vi "launch_automatic.vi"(5 "waitgroup":T5, 7 "references":T3, 8 "error in (no error)":errorcluster, 10 "data":T1, 11 "vi_reference":variant) -> (0 "error out":errorcluster)   [LabVIEW 2015, in "lv-recipe-machine.lvlib"]
uses:
  lv-recipe-machine.lvlib
  <userlib>/antonio-alexander/lv-waitgroup/public/_controls/api_waitgroup.ctl
  public/_controls/references.ctl
  public/_controls/input.ctl
  public/_controls/input_command.ctl
  public/_controls/output.ctl
  public/_controls/data.ctl
  public/_controls/configuration.ctl
  public/_controls/recipe_data.ctl
  public/_controls/mode.ctl
  public/_controls/manual_state.ctl
  public/_controls/automatic_state.ctl
  public/_controls/recipe_step.ctl
  public/_controls/change.ctl
  public/_controls/status.ctl
  _controls/automatic_vi_variant_data.ctl
  public/_controls/vi_reference_automatic_step.ctl
  public/_controls/vi_reference_criteria.ctl
  public/_controls/vi_reference_transition.ctl
  <userlib>/antonio-alexander/lv-waitgroup/lv-waitgroup.lvlib
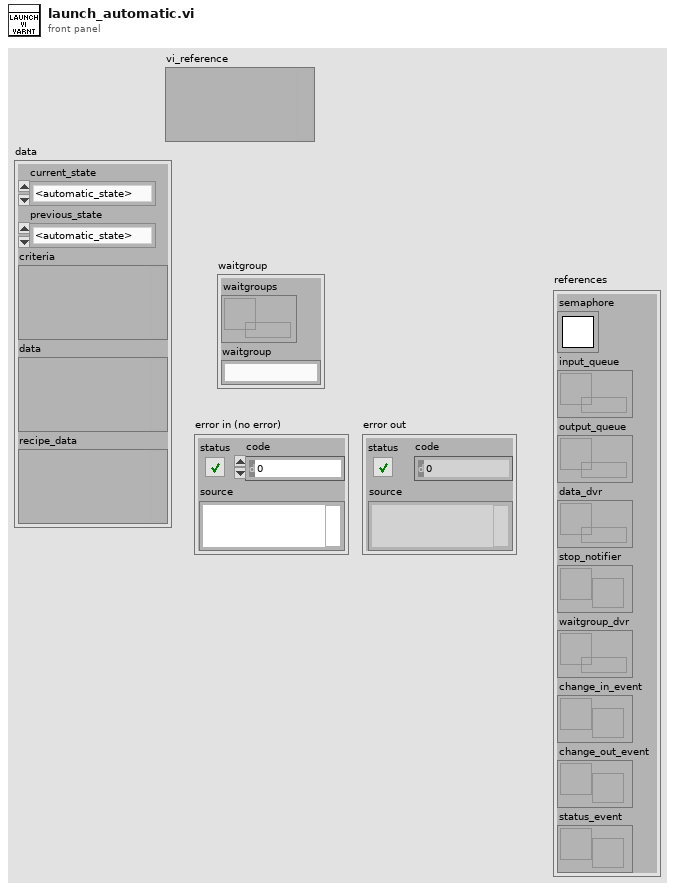
[diagram p1: front panel]
types:
  T1 = typedef "lv-recipe-machine.lvlib/automatic_vi_variant_data.ctl" = cluster{"current_state":T2, "previous_state":T2, "criteria":variant, "data":variant, "recipe_data":variant}
  T2 = typedef "lv-recipe-machine.lvlib/automatic_state.ctl" = enum16{"<automatic_state>", "failed", "idle", "running", "paused", "transition", "stopped", "<null>"}
  T3 = typedef "lv-recipe-machine.lvlib/references.ctl" = cluster{"semaphore":T4, "input_queue":refnum<queue>, "output_queue":refnum<queue>, "data_dvr":refnum<data-value>, "stop_notifier":refnum<notifier>, "waitgroup_dvr":refnum<data-value>, "change_in_event":refnum<user-event>, "change_out_event":refnum<user-event>, "status_event":refnum<user-event>}
  T4 = typedef "Semaphore RefNum" = refnum<k1>
  T5 = typedef "lv-waitgroup.lvlib/api_waitgroup.ctl" = cluster{"waitgroups":refnum<data-value>, "waitgroup":string}
  T6 = typedef "lv-recipe-machine.lvlib/vi_reference_automatic_step.ctl" = refnum<vi>
  T7 = typedef "lv-recipe-machine.lvlib/vi_reference_criteria.ctl" = refnum<vi>
  T8 = typedef "lv-recipe-machine.lvlib/vi_reference_transition.ctl" = refnum<vi>
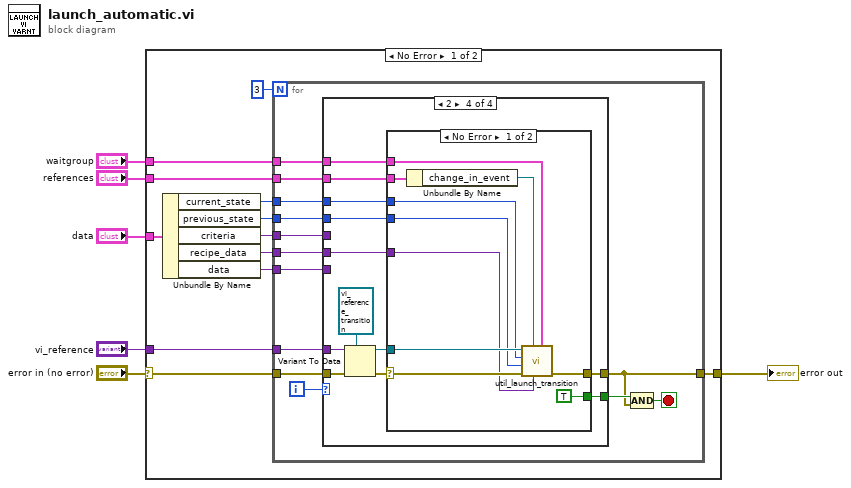
[diagram p0: block diagram]
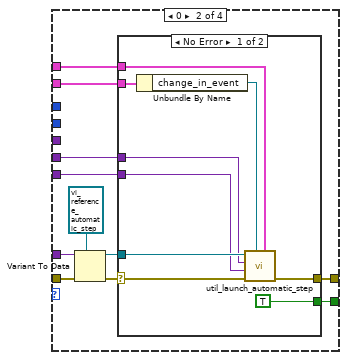
[diagram p3: hidden frame]
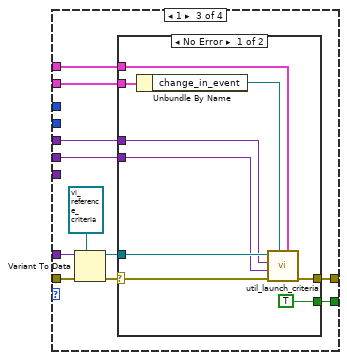
[diagram p5: hidden frame]
diagram:
  n1 = case shown="No Error" "error in (no error)" {
    selector: "error in (no error)" -> [w18 w98]
    tunnel: [w16 w98] -> w5
    tunnel: "waitgroup" -> [w15 _]
    tunnel: "references" -> [w14 _]
    tunnel: "vi_reference" -> [w13 _]
    tunnel: "data" -> [w12 _]
    frame No Error {
      n2 = Unbundle By Name(w12) -> ("current_state"=w11:T2, "previous_state"=w10:T2, "criteria"=w9:variant, "recipe_data"=w8:variant, "data"=w7:variant)
      n3 = for {
        N: 3 -> [_]
        tunnel: w13 -> [w31]
        tunnel: w15 -> [w28]
        tunnel: w14 -> [w27]
        tunnel: w18 -> [w30]
        tunnel: [w25] -> w16
        tunnel: w11 -> [w23]
        tunnel: w10 -> [w22]
        tunnel: w9 -> [w21]
        tunnel: w8 -> [w20]
        tunnel: w7 -> [w19]
        i -> [w29]
        stop <- w24 stop-if-true
        n4 = case shown="2" w29 {
          tunnel: w31 -> [_ w43 w64 w86]
          tunnel: w30 -> [w32 w42 w63 w85]
          tunnel: [w32 w38 w59 w81] -> w25
          tunnel: w28 -> [_ w37 w58 w80]
          tunnel: w27 -> [_ w36 w57 w79]
          tunnel: [_ w35 w56 w78] -> w26
          tunnel: w23 -> [_ _ _ w77]
          tunnel: w22 -> [_ _ _ w76]
          tunnel: w21 -> [_ _ w55 _]
          tunnel: w20 -> [_ w33 w54 w75]
          tunnel: w19 -> [_ w34 _ _]
          frame Default {
          }
          frame 0 {
            n5 = Variant To Data(error in=w42, type=T6 refnum ("vi_reference_step_action"), Variant=w43) -> (data=w39:T6, error out=w40:errorcluster)
            n6 = case shown="No Error" w40 {
              selector: w40 -> [w52 w53]
              tunnel: w39 -> [w51 _]
              tunnel: [w50 w53] -> w38
              tunnel: w37 -> [w49 _]
              tunnel: w36 -> [w48 _]
              tunnel: [TRUE _] -> w35
              tunnel: w34 -> [w44 _]
              tunnel: w33 -> [w45 _]
              frame No Error {
                n7 = Unbundle By Name(w48) -> ("change_in_event"=w47:refnum<user-event>)
                n8 = call "util_launch_automatic_step.vi"("waitgroup"=w49, "change_in_event"=w47, "error in (no error)"=w52, "data"=w44, "recipe_data"=w45, "step_vi_reference"=w51) -> ("error out"=w50:errorcluster)  [unwired: 5 in]
              }
              frame Error {
              }
            }
          }
          frame 1 {
            n9 = Variant To Data(error in=w63, type=T7 refnum ("vi_reference_criteria"), Variant=w64) -> (data=w60:T7, error out=w61:errorcluster)
            n10 = case shown="No Error" w61 {
              selector: w61 -> [w73 w74]
              tunnel: w60 -> [w72 _]
              tunnel: [w71 w74] -> w59
              tunnel: w58 -> [w70 _]
              tunnel: w57 -> [w69 _]
              tunnel: [TRUE _] -> w56
              tunnel: w55 -> [w66 _]
              tunnel: w54 -> [w65 _]
              frame No Error {
                n11 = Unbundle By Name(w69) -> ("change_in_event"=w68:refnum<user-event>)
                n12 = call "util_launch_criteria.vi"("waitgroup"=w70, "change_in_event"=w68, "error in (no error)"=w73, "recipe_data"=w65, "criteria"=w66, "criteria_vi_reference"=w72) -> ("error out"=w71:errorcluster)  [unwired: 5 in]
              }
              frame Error {
              }
            }
          }
          frame 2 {
            n13 = Variant To Data(error in=w85, type=T8 refnum ("vi_reference_transition"), Variant=w86) -> (data=w82:T8, error out=w83:errorcluster)
            n14 = case shown="No Error" w83 {
              selector: w83 -> [w96 w97]
              tunnel: w82 -> [w95 _]
              tunnel: [w94 w97] -> w81
              tunnel: w80 -> [w93 _]
              tunnel: w79 -> [w92 _]
              tunnel: [TRUE _] -> w78
              tunnel: w77 -> [w89 _]
              tunnel: w76 -> [w88 _]
              tunnel: w75 -> [w87 _]
              frame No Error {
                n15 = Unbundle By Name(w92) -> ("change_in_event"=w91:refnum<user-event>)
                n16 = call "util_launch_transition.vi"("waitgroup"=w93, "recipe_data"=w87, "change_in_event"=w91, "error in (no error)"=w96, "previous_state"=w88, "current_state"=w89, "transition_vi_reference"=w95) -> ("error out"=w94:errorcluster)  [unwired: 4 in]
              }
              frame Error {
              }
            }
          }
        }
        n17 = Compound Arithmetic op=AND(w26, w25) -> (w24:bool)
      }
    }
    frame Error {
    }
  }
  "error out" <- w5
